vi "Index Status.vi"() -> ()   [LabVIEW 2021]
uses:
  Controls/Indexing.ctl
panel:
  out "Index Status":T1
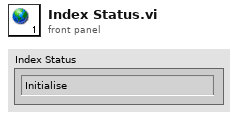
[diagram p1: front panel]
types:
  T1 = typedef "Indexing.ctl" = enum16{"Initialise", "Go CCW", "Go CW (till stopper)", "Go CW (till complete)", "Return CCW", "Done", "Error"}
diagram:
